vi "Msg To.vi"() -> (3 "Setup Msg Strategy out":refnum<class "Setup Msg Strategy.lvclass">)   [LabVIEW 2021, in "jettl.lvlib" / "Setup.lvlib"]
uses:
  Setup.lvlib
  Setup Msg Strategy/Setup Msg Strategy.lvclass
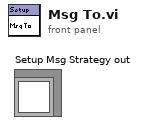
[diagram p1: front panel]
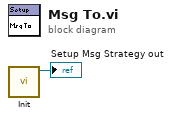
[diagram p0: block diagram]
diagram:
  n1 = call "Init.vi"() -> ("Setup Msg Strategy out"=→"Setup Msg Strategy out":refnum<class "Setup Msg Strategy.lvclass">)  [unwired: 11 in]
